vi "Read I16.vi"(8 "error in":errorcluster, 9 "RegisterOffset":u32, 10 "register name":string, 11 "session in":u32) -> (0 "error out":errorcluster, 2 "value out":i16, 3 "session out":u32)   [LabVIEW 2024, in "FPGA Register IO.lvlib"]
uses:
  FPGA Register IO.lvlib
  NiFpga.dll
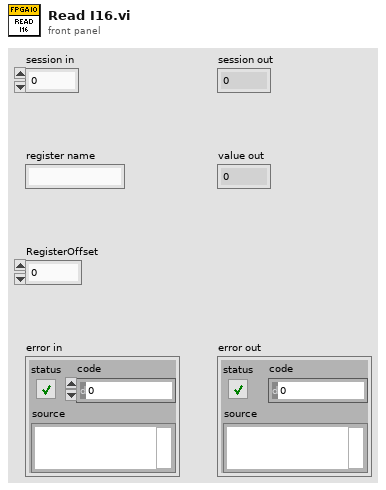
[diagram p1: front panel]
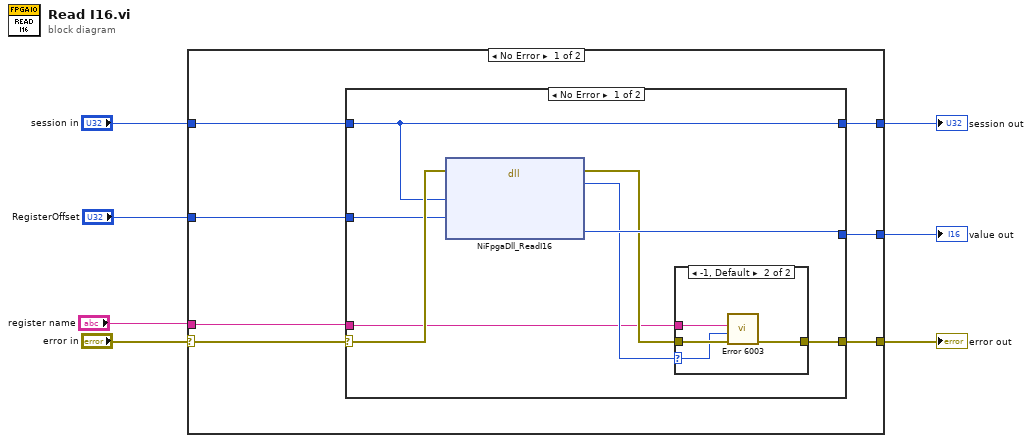
[diagram p0: block diagram]
diagram:
  n1 = case shown="No Error" "error in" {
    selector: "error in" -> [w9 w30]
    tunnel: [w14 w30] -> w7
    tunnel: [w13 _] -> w6
    tunnel: [w12 w31] -> w5
    tunnel: "session in" -> [w10 w31]
    tunnel: "register name" -> [w11 _]
    tunnel: "RegisterOffset" -> [w8 _]
    frame No Error {
      n2 = case shown="No Error" w9 {
        selector: w9 -> [w21 w29]
        tunnel: w10 -> [w20 w28]
        tunnel: [w19 w29] -> w14
        tunnel: [w22 _] -> w13
        tunnel: [w20 w28] -> w12
        tunnel: w11 -> [w16 _]
        tunnel: w8 -> [w15 _]
        frame No Error {
          n3 = dll-call lib="NiFpga.*" fn="NiFpgaDll_ReadI16"(error in=w21, "session"=w20, "offset"=w15) -> (error out=w18:errorcluster, "status"=w17:i32, "value"=w22:i16)  [unwired: 5 in, 1 out]
          n4 = case shown="-1, Default" w17 {
            selector: w17 -> [_ w24]
            tunnel: w18 -> [w23 w27]
            tunnel: [w23 w26] -> w19
            tunnel: w16 -> [_ w25]
            frame 0 {
            }
            frame -1, Default {
              n5 = call "Error 6003.vi"("error in (no error)"=w27, "rio status code"=w24, "register name"=w25) -> ("error out"=w26:errorcluster)  [unwired: 8 in]
            }
          }
        }
        frame Error {
        }
      }
    }
    frame Error {
    }
  }
  "error out" <- w7
  "session out" <- w5
  "value out" <- w6
